vi "BlendAlphaWithBg.vi"(5 "Remove Mask? (T)":bool=TRUE, 7 "Parallel Instances (1)":i32=1, 10 "Background Color (White)":u32(colorbox)=16777215, 11 "Image In":T1) -> (3 "Image Out":T1)   [LabVIEW 2020, in "lv-image.lvlib"]
doc: "Perform Alpha Blending (https://fr.wikipedia.org/wiki/Alpha_blending) with the background color.\nBackground color Alpha channel is ignored.\n\nBy default, removes image mask since we don't need it (we're using alpha).\n\nWire <B>Parallel Instances</B> to set a number of parallel instances to speed up computation. 4 works good.\n<B>Be carefull not nesting parallel loops though!</B> That's why I've set it to 1."
uses:
  lv-image.lvlib
  <vilib>/picture/picture.llb/imagedata.ctl
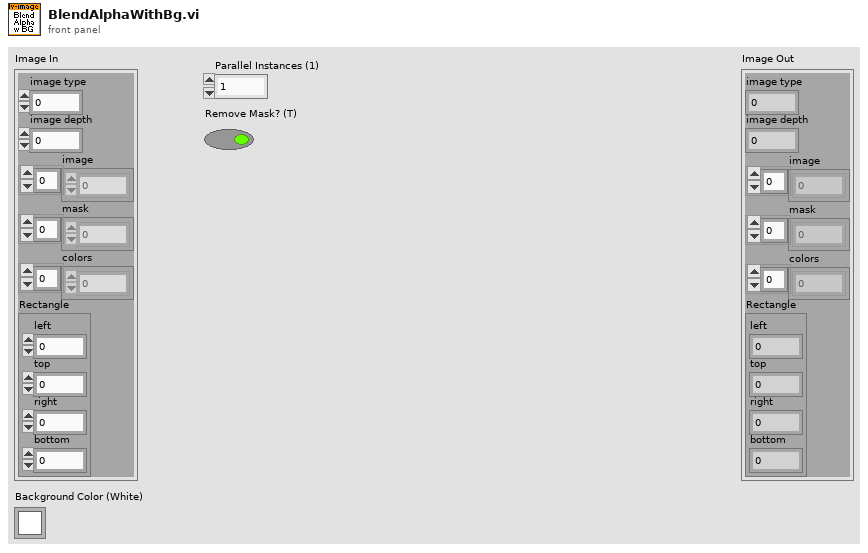
[diagram p1: front panel]
types:
  T1 = typedef "imagedata.ctl" = cluster{"image type":i32, "image depth":i32, "image":u8[], "mask":u8[], "colors":u32[], "Rectangle":cluster{"left":i16, "top":i16, "right":i16, "bottom":i16}}
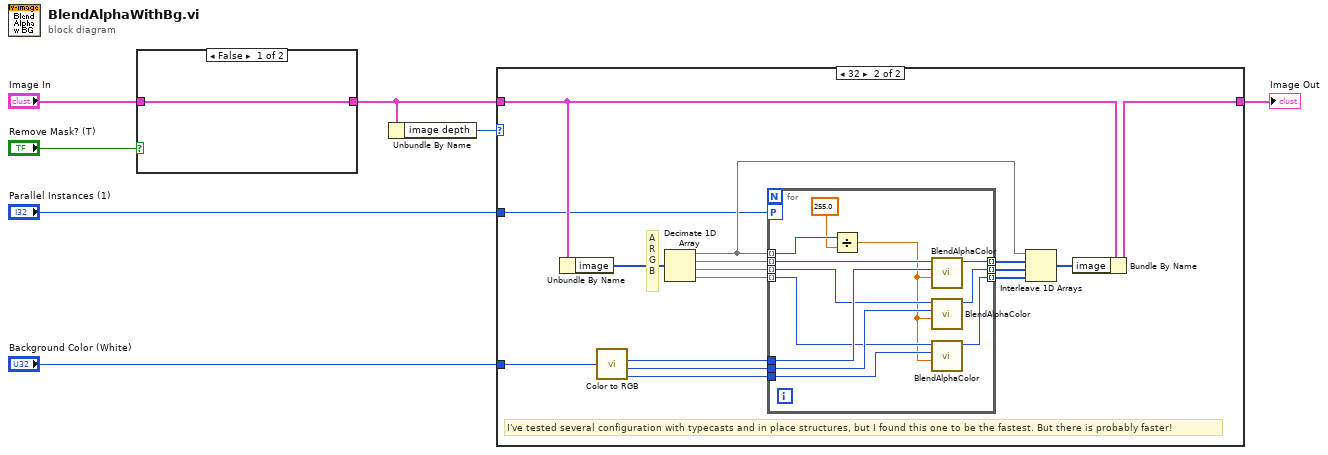
[diagram p0: block diagram]
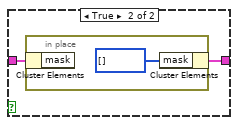
[diagram p2: hidden frame]
diagram:
  n1 = case shown="False" "Remove Mask? (T)" {
    tunnel: "Image In" -> [w8 w10]
    tunnel: [w8 w9] -> w2
    frame False {
    }
    frame True {
      n2 = in-place {
        n3 = in-place-cluster #1(w10) -> ()  [unwired: 1 out]
        n4 = in-place-cluster #1("mask"=u8[] []) -> (w9:T1)
      }
    }
  }
  n5 = Unbundle By Name(w2) -> ("image depth"=w7:i32)
  n6 = case shown="32" w7 {
    tunnel: "Background Color (White)" -> [_ w28]
    tunnel: w2 -> [w12 w16]
    tunnel: [w12 w14] -> w5
    tunnel: "Parallel Instances (1)" -> [_ w13]
    frame Default {
    }
    frame 32 {
      # "I've tested several configuration with typecasts and in place structures, but I found this one to be the fastest. But there is probably faster!"
      # "A\nR\nG\nB"
      n7 = Unbundle By Name(w16) -> ("image"=w27:u8[])
      n8 = call <vilib>:"Color to RGB.vi"("Color"=w28) -> ("R"=w23:u8, "G"=w22:u8, "B"=w21:u8)  [unwired: 1 out]
      n9 = Decimate 1D Array(w27) -> (w20:u8[], w26:u8[], w25:u8[], w24:u8[])
      n10 = for {
        tunnel: w20 -> [w40] mode=indexing
        tunnel: w26 -> [w38] mode=indexing
        tunnel: w25 -> [w36] mode=indexing
        tunnel: w24 -> [w34] mode=indexing
        tunnel: w23 -> [w37]
        tunnel: w22 -> [w35]
        tunnel: w21 -> [w33]
        tunnel: [w32] -> w19 mode=indexing
        tunnel: [w31] -> w18 mode=indexing
        tunnel: [w30] -> w17 mode=indexing
        workers-P: w13 -> [_]
        n11 = Divide(x=w40, y=255.0) -> (x/y=w29:dbl)
        n12 = call "BlendAlphaColor.vi"("Alpha [0..1]"=w29, "BG Color Component"=w37, "Image Color Component"=w38) -> ("New Image Color"=w32:u8)  [unwired: 8 in]
        n13 = call "BlendAlphaColor.vi"("Alpha [0..1]"=w29, "BG Color Component"=w35, "Image Color Component"=w36) -> ("New Image Color"=w31:u8)  [unwired: 8 in]
        n14 = call "BlendAlphaColor.vi"("Alpha [0..1]"=w29, "BG Color Component"=w33, "Image Color Component"=w34) -> ("New Image Color"=w30:u8)  [unwired: 8 in]
      }
      n15 = Interleave 1D Arrays(w20, w19, w18, w17) -> (w15:u8[])
      n16 = Bundle By Name(cluster=w16, "image"=w15) -> (w14:T1)
    }
  }
  "Image Out" <- w5
